vi "KB-外环4相位选点.vi"(11 "外环3D":dbl[][](array[numeric])) -> (0 "添加的数组":dbl[](array[numeric]), 2 "高度差":dbl, 3 "外环平均高度值":dbl)   [LabVIEW 2015]
uses:
  <vilib>/Math Plots/3D Math Plots/3D Surface/3D Surface XCtrl/3D Surface.xctl
  <vilib>/Math Plots/3D Math Plots/3D Surface/3D Surface Datatype/Public/Plot Helper (Matrix).vi
  <vilib>/Math Plots/3D Math Plots/3D Surface/3D Surface Datatype/3D Surface Datatype.lvclass
panel:
  out "x/y":dbl
  out "中心行前半部波形图 2":dbl[](graph)
  out "Filtered Signal 3":dbl[](graph) caption="滤波后的信号"
  out "中心行 3":dbl[](array[numeric])
  out "Filtered Signal 2":dbl[](graph) caption="滤波后的信号"
  out "Filtered Signal":dynamicdata(graph) caption="滤波后的信号"
  out "中心行 2":dbl[](array[numeric])
  out "数组 2":dbl[](array[numeric])
  out "数组":dbl[](array[numeric])
  out "外环3D 2":dbl[][](array[numeric])
  out "列 后半部平均高度":dbl
  out "列 前半部平均高度":dbl
  out "后半部平均高度":dbl
  out "前半部平均高度":dbl
  out "中心行后半部波形图":dbl[](graph)
  out "中心行前半部波形图":dbl[](graph)
  out "中心行半径":dbl
  out "中心列":dbl[](array[numeric])
  out "中心行":dbl[](array[numeric])
  out "中心列波形":dbl[](graph)
  out "中心列波形图":dbl[](graph)
  out "大小":i32[](array[numeric])
  out "外环":refnum<class "3D Plot Datatype.lvclass">[](xcontrol)
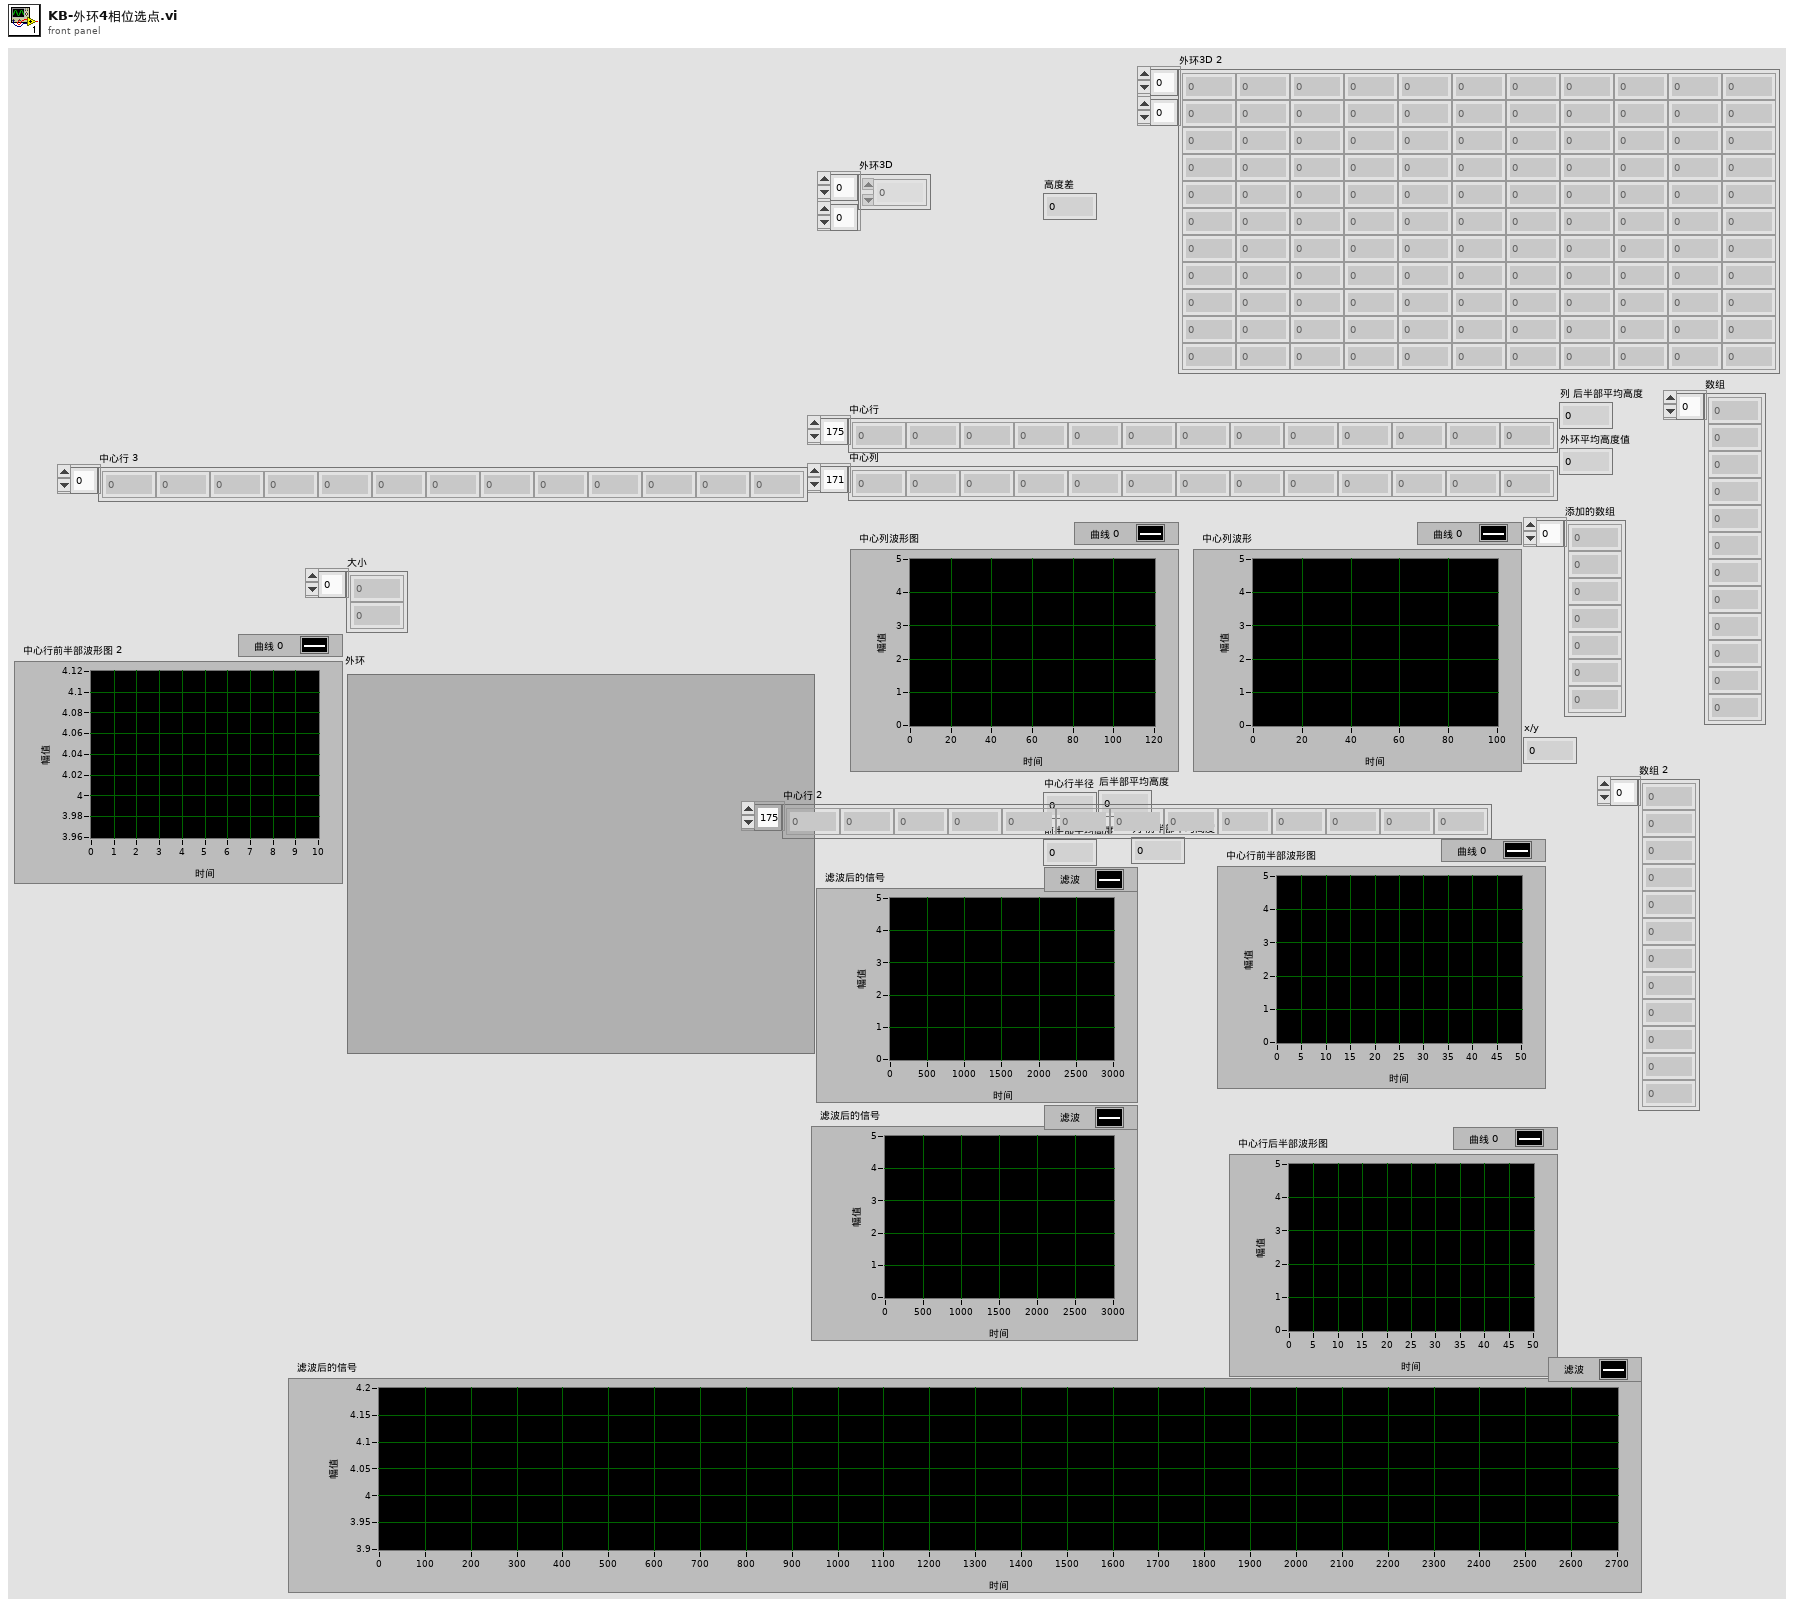
[diagram p1: front panel]
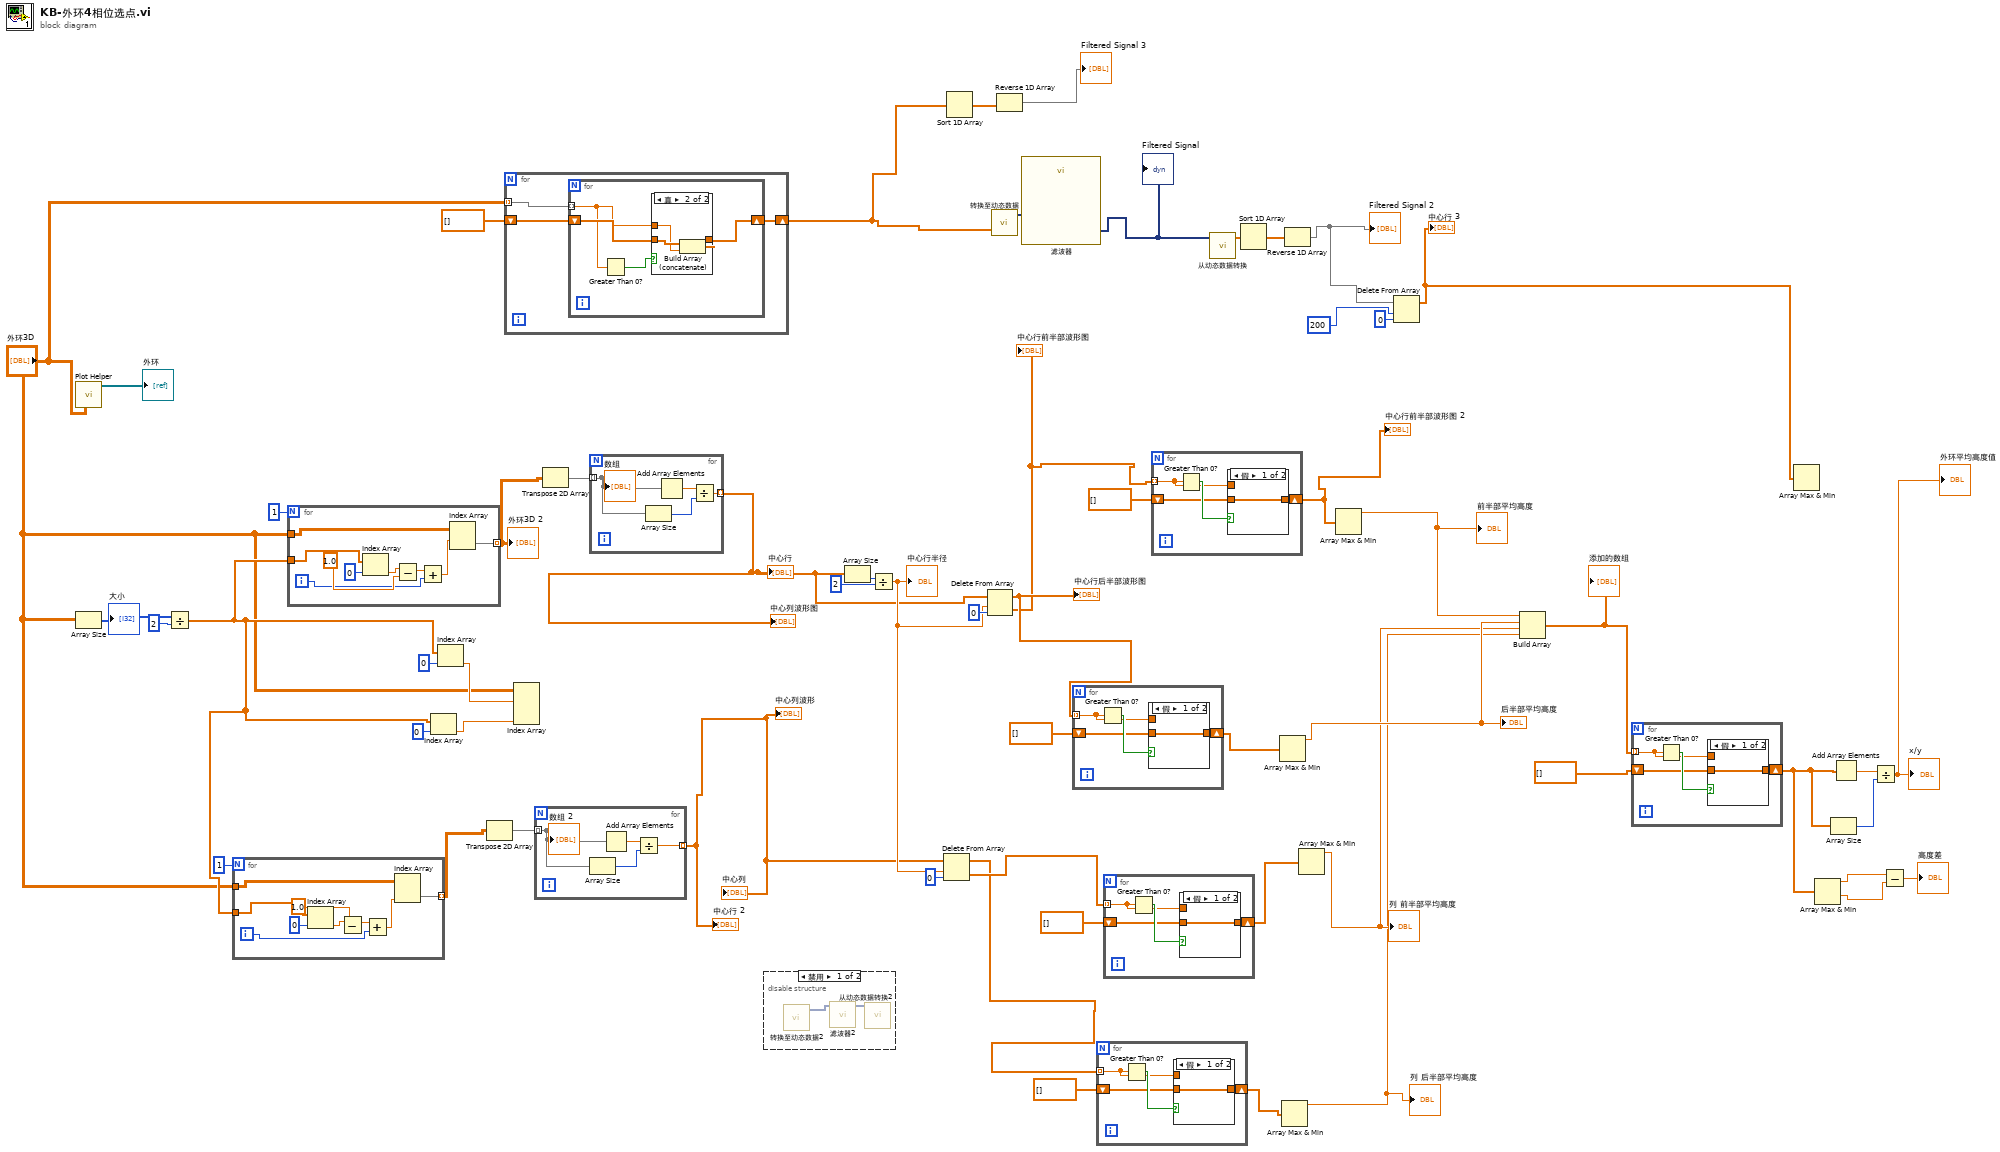
[diagram p0: block diagram]
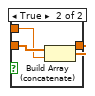
[diagram p4: hidden frame]
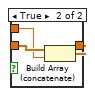
[diagram p5: hidden frame]
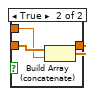
[diagram p6: hidden frame]
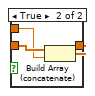
[diagram p7: hidden frame]
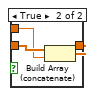
[diagram p8: hidden frame]
diagram:
  n1 = call-poly <vilib>:"Plot Helper.vi"("z matrix"="外环3D") -> ("3D Plot lvclass Array out"=→"外环":refnum<class "3D Plot Datatype.lvclass">[])  [unwired: 5 in, 5 out]
  n2 = Array Size(array="外环3D") -> (size(s)=w58:i32[])
  "大小" <- w58
  n3 = Divide(x=w58, y=2) -> (x/y=w28:dbl[])
  n4 = for {
    N: 1 -> [_]
    tunnel: "外环3D" -> [w62]
    tunnel: w28 -> [w67]
    tunnel: [w61] -> w30 mode=indexing
    i -> [w63]
    n5 = Index Array(array=w67, index=0 ("索引")) -> (element=w66:dbl)
    n6 = Subtract(x=w66, y=1.0) -> (x-y=w64:dbl)
    n7 = Add(x=w64, y=w63) -> (x+y=w60:dbl)
    n8 = Index Array(array=w62, index (col)=w60) -> (element=w61:dbl[])  [unwired: 1 in]
  }
  n9 = for {
    N: 1 -> [_]
    tunnel: "外环3D" -> [w71]
    tunnel: w28 -> [w76]
    tunnel: [w69] -> w34 mode=indexing
    i -> [w72]
    n10 = Index Array(array=w76, index=0 ("索引")) -> (element=w75:dbl)
    n11 = Subtract(x=w75, y=1.0) -> (x-y=w73:dbl)
    n12 = Add(x=w73, y=w72) -> (x+y=w70:dbl)
    n13 = Index Array(array=w71, index (row)=w70) -> (element=w69:dbl[])  [unwired: 1 in]
  }
  "外环3D 2" <- w34
  n14 = Index Array(array=w28, index=0 ("索引")) -> (element=w53:dbl)
  n15 = Index Array(array=w28, index=0 ("索引")) -> (element=w55:dbl)
  n16 = Transpose 2D Array(2D array=w30) -> (transposed array=w31:dbl[][])
  n17 = for {
    shift-right: [w78] -> w16
    shift-left: dbl[] [] -> [w80]
    tunnel: "外环3D" -> [w79] mode=indexing
    n18 = for {
      tunnel: w79 -> [w82] mode=indexing
      shift-right: [w83] -> w78
      shift-left: w80 -> [w84]
      n19 = Greater Than 0?(x=w82) -> (x > 0?=w81:bool)
      n20 = case shown="真" w81 {
        tunnel: w84 -> [w85 w88]
        tunnel: w82 -> [_ w87]
        tunnel: [w85 w86] -> w83
        frame False {
        }
        frame True {
          n21 = Build Array (concatenate)(w88, w87) -> (w86:dbl[])
        }
      }
    }
  }
  n22 = Index Array(array="外环3D", index (row) #1=w55, index (col) #2=w53) -> ()  [unwired: 2 in, 2 out]
  n23 = for {
    tunnel: w31 -> [w92] mode=indexing
    tunnel: [w89] -> w27 mode=indexing
    n24 = Array Size(array=w92) -> (size(s)=w90:i32)
    n25 = Add Array Elements(numeric array=w92) -> (sum=w91:dbl)
    n26 = Divide(x=w91, y=w90) -> (x/y=w89:dbl)
    "数组 2" <- w92
  }
  "中心列波形" <- w27
  "中心列" <- w27
  "中心行 2" <- w27
  n27 = Transpose 2D Array(2D array=w34) -> (transposed array=w33:dbl[][])
  n28 = for {
    tunnel: w33 -> [w96] mode=indexing
    tunnel: [w93] -> w32 mode=indexing
    n29 = Array Size(array=w96) -> (size(s)=w94:i32)
    n30 = Add Array Elements(numeric array=w96) -> (sum=w95:dbl)
    n31 = Divide(x=w95, y=w94) -> (x/y=w93:dbl)
    "数组" <- w96
  }
  "中心列波形图" <- w32
  "中心行" <- w32
  n32 = disable-structure shown="禁用" {
    frame Disabled {
      n33 = call "转换至动态数据2"() -> ("Dynamic Data Type"=w97:dynamicdata)  [unwired: 4 in]
      n34 = call "滤波器2"("Signal"=w97) -> ("Filtered Signal"=w98:dynamicdata)  [unwired: 9 in, 1 out]
      n35 = call "从动态数据转换2"("Dynamic Data Type"=w98) -> ()  [unwired: 3 in, 1 out]
    }
    frame Enabled {
    }
  }
  n36 = Array Size(array=w32) -> (size(s)=w52:i32)
  n37 = Divide(x=w52, y=2) -> (x/y=w45:dbl)
  "中心行半径" <- w45
  n38 = Delete From Array(array=w27, length=w45, index=0 ("索引")) -> (deleted portion=w3:dbl[], array with subset deleted=w1:dbl[])
  n39 = Sort 1D Array(array=w16) -> (sorted array=w15:dbl[])
  n40 = Delete From Array(array=w32, length=w45, index=0 ("索引")) -> (deleted portion=w2:dbl[], array with subset deleted=w4:dbl[])
  "中心行前半部波形图" <- w2
  "中心行后半部波形图" <- w4
  n41 = call "转换至动态数据"("Array"=w16) -> ("Dynamic Data Type"=w24:dynamicdata)  [unwired: 3 in]
  n42 = Reverse 1D Array(array=w15) -> (reversed array=→"Filtered Signal 3":dbl[])
  n43 = call "滤波器"("Signal"=w24) -> ("Filtered Signal"=w23:dynamicdata)  [unwired: 9 in, 1 out]
  "Filtered Signal" <- w23
  n44 = for {
    shift-right: [w99] -> w11
    shift-left: dbl[] [] -> [w101]
    tunnel: w4 -> [w100] mode=indexing
    n45 = Greater Than 0?(x=w100) -> (x > 0?=w102:bool)
    n46 = case shown="假" w102 {
      tunnel: w101 -> [w103 w106]
      tunnel: w100 -> [_ w105]
      tunnel: [w103 w104] -> w99
      frame False {
      }
      frame True {
        n47 = Build Array (concatenate)(w106, w105) -> (w104:dbl[])
      }
    }
  }
  n48 = for {
    shift-right: [w107] -> w7
    shift-left: dbl[] [] -> [w109]
    tunnel: w1 -> [w108] mode=indexing
    n49 = Greater Than 0?(x=w108) -> (x > 0?=w110:bool)
    n50 = case shown="假" w110 {
      tunnel: w109 -> [w111 w114]
      tunnel: w108 -> [_ w113]
      tunnel: [w111 w112] -> w107
      frame False {
      }
      frame True {
        n51 = Build Array (concatenate)(w114, w113) -> (w112:dbl[])
      }
    }
  }
  n52 = for {
    shift-right: [w115] -> w9
    shift-left: dbl[] [] -> [w117]
    tunnel: w3 -> [w116] mode=indexing
    n53 = Greater Than 0?(x=w116) -> (x > 0?=w118:bool)
    n54 = case shown="假" w118 {
      tunnel: w117 -> [w119 w122]
      tunnel: w116 -> [_ w121]
      tunnel: [w119 w120] -> w115
      frame False {
      }
      frame True {
        n55 = Build Array (concatenate)(w122, w121) -> (w120:dbl[])
      }
    }
  }
  n56 = for {
    shift-right: [w123] -> w13
    shift-left: dbl[] [] -> [w125]
    tunnel: w2 -> [w124] mode=indexing
    n57 = Greater Than 0?(x=w124) -> (x > 0?=w126:bool)
    n58 = case shown="假" w126 {
      tunnel: w125 -> [w127 w130]
      tunnel: w124 -> [_ w129]
      tunnel: [w127 w128] -> w123
      frame False {
      }
      frame True {
        n59 = Build Array (concatenate)(w130, w129) -> (w128:dbl[])
      }
    }
  }
  "中心行前半部波形图 2" <- w13
  n60 = call "从动态数据转换"("Dynamic Data Type"=w23) -> ("Array"=w22:dbl[])  [unwired: 3 in]
  n61 = Sort 1D Array(array=w22) -> (sorted array=w21:dbl[])
  n62 = Array Max & Min(array=w11) -> (max value=w10:dbl)  [unwired: 3 out]
  "后半部平均高度" <- w10
  n63 = Array Max & Min(array=w7) -> (max value=w6:dbl)  [unwired: 3 out]
  "列 后半部平均高度" <- w6
  n64 = Reverse 1D Array(array=w21) -> (reversed array=w20:dbl[])
  "Filtered Signal 2" <- w20
  n65 = Array Max & Min(array=w9) -> (max value=w8:dbl)  [unwired: 3 out]
  "列 前半部平均高度" <- w8
  n66 = Array Max & Min(array=w13) -> (max value=w12:dbl)  [unwired: 3 out]
  "前半部平均高度" <- w12
  n67 = Delete From Array(array=w20, length=200 ("索引"), index=0 ("索引")) -> (array with subset deleted=w19:dbl[])  [unwired: 1 out]
  "中心行 3" <- w19
  n68 = Build Array(w12, w10, w8, w6) -> (w42:dbl[])
  "添加的数组" <- w42
  n69 = for {
    shift-right: [w131] -> w39
    shift-left: dbl[] [] -> [w133]
    tunnel: w42 -> [w132] mode=indexing
    n70 = Greater Than 0?(x=w132) -> (x > 0?=w134:bool)
    n71 = case shown="假" w134 {
      tunnel: w133 -> [w135 w138]
      tunnel: w132 -> [_ w137]
      tunnel: [w135 w136] -> w131
      frame False {
      }
      frame True {
        n72 = Build Array (concatenate)(w138, w137) -> (w136:dbl[])
      }
    }
  }
  n73 = Array Max & Min(array=w19) -> ()  [unwired: 4 out]
  n74 = Array Max & Min(array=w39) -> (max value=w38:dbl, min value=w37:dbl)  [unwired: 2 out]
  n75 = Array Size(array=w39) -> (size(s)=w40:i32)
  n76 = Add Array Elements(numeric array=w39) -> (sum=w41:dbl)
  n77 = Divide(x=w41, y=w40) -> (x/y=→"外环平均高度值" →"x/y":dbl)
  n78 = Subtract(x=w38, y=w37) -> (x-y=→"高度差":dbl)
